vi "EXA_acceptCommand_Example.vi"(8 "error in (no error)":errorcluster, 11 "command_Example_Ctl":T1) -> (0 "error out":errorcluster, 2 "function return":i32, 3 "command_Example_Ctl out":T1)   [LabVIEW 2016, in "SALLV_EXA.lvlib"]
doc: "int EXA_shm_acceptCommand_ExampleLV(EXA_command_ExampleLV *command_Example_Ctl );"
uses:
  SALLV_EXA.lvlib
  DataTypes/command_Example.ctl
  SALLV_EXA.so
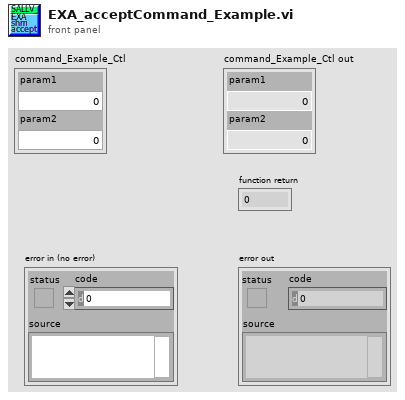
[diagram p1: front panel]
types:
  T1 = typedef "SALLV_EXA.lvlib/command_Example.ctl" = cluster{"param1":dbl, "param2":dbl}
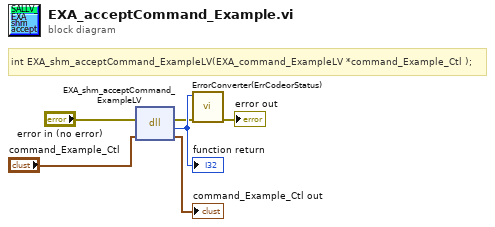
[diagram p0: block diagram]
diagram:
  # "int EXA_shm_acceptCommand_ExampleLV(EXA_command_ExampleLV *command_Example_Ctl );"
  n1 = dll-call lib="home/andres/Desktop/EXA_SAL_LV/SALLV_EXA.*" fn="EXA_shm_acceptCommand_ExampleLV"(error in="error in (no error)", "command_Example_Ctl"="command_Example_Ctl") -> (error out=w2:errorcluster, w6:i32, "command_Example_Ctl"=→"command_Example_Ctl out":T1)  [unwired: 2 in, 1 out]
  "function return" <- w6
  n2 = call "ErrorConverter(ErrCodeorStatus).vi"("error in (no error)"=w2, "error code"=w6) -> ("error out"=→"error out":errorcluster)  [unwired: 9 in]
